vi "ERRMSG.VI"(0 "ErrCode":i32) -> (1 "ErrMsg":string, 2 "ErrCode (Out)":i32)   [LabVIEW 2010]
doc: "Returns the error message associated with an error code."
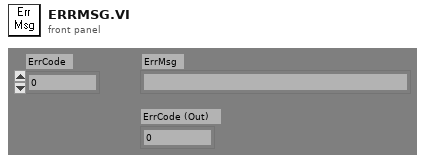
[diagram p1: front panel]
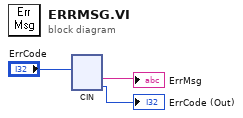
[diagram p0: block diagram]
diagram:
  n1 = cin("ErrCode") -> (→"ErrMsg":string, →"ErrCode (Out)":i32)  [unwired: 3 in]
